vi "201541062019.vi"() -> ()   [LabVIEW 2017]
panel:
  out "?":bool
  out "倒计时":string
  in  "开始倒计时":bool
  in  "定时时间选择":enum16{"6秒", "10秒", "20秒"}(ring)
  in  "停止":bool
  # "倒 计 时 器"
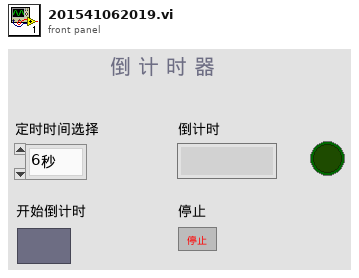
[diagram p1: front panel]
types:
  T1 = enum8{"Enabled", "Disabled", "Disabled and Grayed Out"}
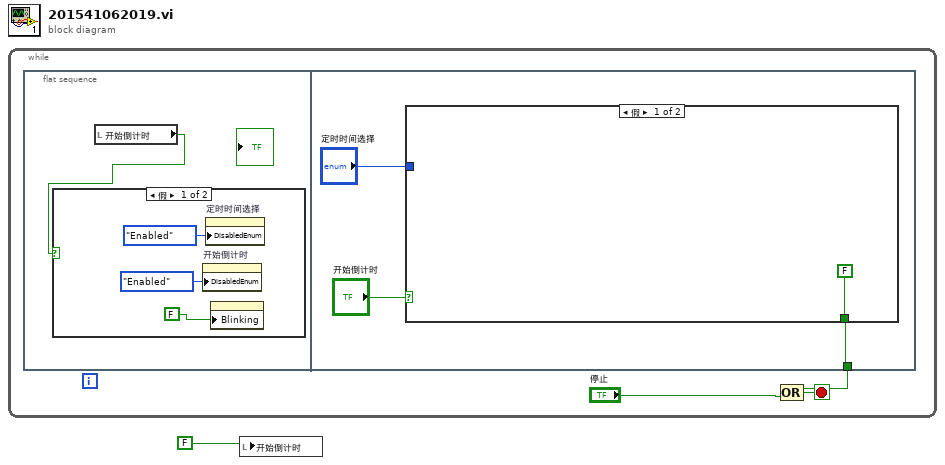
[diagram p0: block diagram]
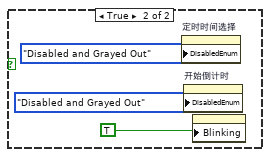
[diagram p2: hidden frame]
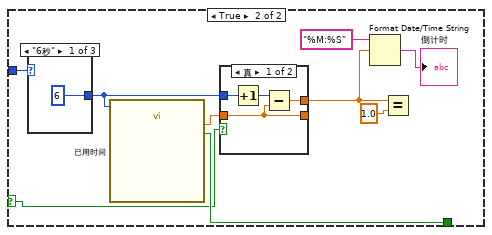
[diagram p3: hidden frame]
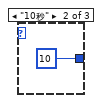
[diagram p5: hidden frame]
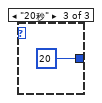
[diagram p6: hidden frame]
diagram:
  n1 = while {
    stop <- w3 stop-if-true
    n2 = flat-sequence {
      tunnel: [w12] -> w2
      frame #0 {
        n3 = local read "开始倒计时"() -> (w5:bool)
        n4 = case shown="假" w5 {
          frame False {
            n5 = property on="开始倒计时" class="Bool (严格)"("DisabledEnum"=T1."Enabled" ("禁用")) -> ()  [unwired: 2 in, 2 out]
            n6 = property on="定时时间选择" class="Enum (严格)"("DisabledEnum"=T1."Enabled" ("禁用")) -> ()  [unwired: 2 in, 2 out]
            n7 = property class="Bool (严格)"("Blinking"=FALSE) -> ()  [unwired: 2 in, 2 out]
          }
          frame True {
            n8 = property on="定时时间选择" class="Enum (严格)"("DisabledEnum"=T1."Disabled and Grayed Out" ("禁用")) -> ()  [unwired: 2 in, 2 out]
            n9 = property on="开始倒计时" class="Bool (严格)"("DisabledEnum"=T1."Disabled and Grayed Out" ("禁用")) -> ()  [unwired: 2 in, 2 out]
            n10 = property class="Bool (严格)"("Blinking"=TRUE) -> ()  [unwired: 2 in, 2 out]
          }
        }
      }
      frame #1 {
        n11 = case shown="假" "开始倒计时" {
          selector: "开始倒计时" -> [_ w19]
          tunnel: "定时时间选择" -> [_ w24]
          tunnel: [FALSE w20] -> w12
          frame False {
          }
          frame True {
            n12 = case shown="\"6秒\"" w24 {
              tunnel: [6 10 20] -> w23
              frame "6秒" {
              }
              frame "10秒" {
              }
              frame "20秒" {
              }
            }
            n13 = call "已用时间"("Time Target (s)"=w23) -> ("Elapsed Time (s)"=w22:dbl, "Time has Elapsed"=w20:bool)  [unwired: 11 in, 6 out]
            n14 = case shown="真" w19 {
              tunnel: w23 -> [w25 _]
              tunnel: w22 -> [w28 w29]
              tunnel: [w28 w29] -> _
              tunnel: [w27 w29] -> w17
              frame True {
                n15 = Increment(x=w25) -> (x+1=w26:i32)
                n16 = Subtract(x=w26, y=w28) -> (x-y=w27:dbl)
              }
              frame False {
              }
            }
            n17 = Format Date/Time String(time format string (%c)="%M:%S", seconds (now)=w17) -> (date/time string=→"倒计时":string)  [unwired: 1 in]
            n18 = Equal?(x=w17, y=1.0) -> ()  [unwired: 1 out]
          }
        }
      }
    }
    n19 = Compound Arithmetic op=OR(w2, "停止") -> (w3:bool)
  }
  n20 = local write "开始倒计时"(FALSE) -> ()
